vi "PH_Beamline.PC _Picture Condition Services.vi"(0 "i ref in":refnum<vi>, 2 "Instancename":string, 3 "No Link?":bool, 5 "error IO":errorcluster) -> (14 "i ref out":refnum<vi>, 19 "error out":errorcluster)   [LabVIEW 2014, in "PH_Beamline.lvlib"]
doc: "This is a Proc Case of the Beamline Class."
uses:
  PH_Beamline.lvlib
  PH_Beamline.Switch+6P Instances.ctl
  PH_Basics/PH_Common/Picture/PH_Picture.Alignment.ctl
  PH_Basics/PH_Common/Picture/PH_Picture.Size.ctl
  CS_Core/CSSystem/CSSystemLib/CSSystemLib.lvlib
  PH_Basics/PH_Beamline_Common/PH_Beamline_Common.lvlib
  PH_Basics/PH_Common/PH_Common.lvlib
  PH_BL-Master/PH_BL-Master.lvlib
panel:
  in  "Switch and 6P Instances":T1="MA01_CH1"
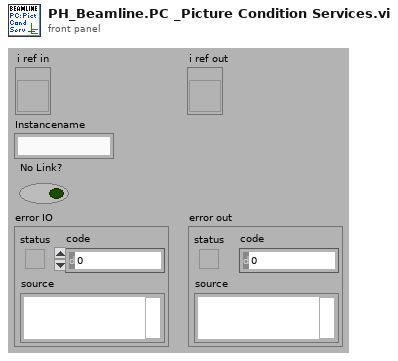
[diagram p1: front panel]
types:
  T1 = typedef "PH_Beamline.lvlib/PH_Beamline.Switch+6P Instances.ctl" = string
  T2 = typedef "PH_BL-Master.lvlib/PH_BL-Master.i attribute.ctl" = cluster{"Remote controlled":bool, "Boolean Condition Service Subscriber":refnum<vi>[], "Picture Condition Service Subscriber":refnum<vi>[], "R2S":cluster{"GUI Ref":refnum<vi>, "State":bool}, "Vacua":cluster{"GUI Ref":refnum<vi>, "Limit":dbl, "Curr Value":dbl, "in range":bool}[], "O2 Inspection":cluster{"GUI Ref":refnum<vi>, "Concentration":dbl, "State":T3}[], "Boolean Status Service Subscriber":cluster{"GUI Ref":refnum<vi>, "Status":T3, "no Link?":bool, "Status Subscriber Class":T4}[], "Picture Status Service Subscriber":cluster{"GUI Ref":refnum<vi>, "Status":T3, "no Link?":bool, "Status Subscriber Class":T4}[], "6P 4Q Service Subscriber":cluster{"GUI Ref":refnum<vi>, "Selector":T5, "no Link?":bool}[], "Index of latest 6P 4Q changing Instance":i32, "Index of latest Picture Status changing Instance":i32, "Index of latest Boolean Status changing Instance":i32, "Vision ID on same Node":string, "Start Phase over?":bool, "GUI Ref Delete":refnum<vi>}
  T3 = typedef "PH_StatusHandler.lvlib/PH_StatusHandler.Status.ctl" = i16
  T4 = typedef "PH_BL-Master.lvlib/PH_BL-Master.Status Subscriber Class.ctl" = enum16{"unknown", "Switch", "BB", "6P Switch", "Switch GUI", "Switch and 6P State", "Force Sensor"}
  T5 = typedef "PH_4_Pos_Selector.lvlib/PH_4_Pos_Selector.Position Selector.ctl" = u16
  T6 = typedef "PH_Common.lvlib/PH_Picture.Alignment.ctl" = enum16{"neutral", "left", "right", "up", "down", "vertical", "horizontal", "left down to right up", "left up to right down"}
  T7 = typedef "PH_Common.lvlib/PH_Picture.Size.ctl" = enum16{"36x36", "48x48", "24x36", "36x24", "12x60", "60x12"}
  T8 = typedef "PH_Beamline.lvlib/PH_Beamline.i attribute.ctl" = cluster{"GUI Refs":cluster{"PA ok":refnum<vi>, "MA ok":refnum<vi>, "fs FE ok":refnum<vi>, "ns FE ok":refnum<vi>, "PA ED ok":refnum<vi>, "MAS ok":refnum<vi>, "Booster ok":refnum<vi>, "Mirrortower ok":refnum<vi>, "In.-Box ok":refnum<vi>, "Compressor ok":refnum<vi>, "Experiment LB ok":refnum<vi>, "Experiment LL ok":refnum<vi>, "PHELIX_Beckhoff_Watchdog":refnum<vi>, "Shutters closed":refnum<vi>, "uOPA ok":refnum<vi>, "Vacuum no shotcond Comp LB":refnum<vi>}, "Refs BL MA":refnum<vi>[], "Refs BL MA-IB":refnum<vi>[], "Refs BL fs":refnum<vi>[], "Refs BL PA ED":refnum<vi>[], "Refs BL MAS":refnum<vi>[], "Refs BL Boo":refnum<vi>[], "Refs BL ns":refnum<vi>[], "Refs BL Mirrortower":refnum<vi>[], "Refs BL Compressor":refnum<vi>[], "Refs BL Exp LB":refnum<vi>[], "Radiation Safety":cluster{"Exp Laserbay":cluster{"Ref Op Mode":refnum<vi>, "Ref Laserbay evacuated":refnum<vi>, "Tagname LB evacuated":string, "Shot Mode":T9, "Laserbay evacuated?":i32, "Tagname HV room locked":string, "HV room locked?":i32, "Ref HV room locked":refnum<vi>, "Tagname bridged?":string, "Ref Bridge":refnum<vi>, "I<1E18W/cm²":bool}, "Exp Laserlab":cluster{"Ref Op Mode":refnum<vi>, "Ref Laserlab evacuated":refnum<vi>, "Tagname LL evacuated":string, "Shot Mode":T9, "Laserlab evacuated?":i32, "Tagname bridged?":string, "Ref Bridge":refnum<vi>, "I<1E18W/cm²":bool}}, "Refs BL LL":refnum<vi>[], "PP Igni Heating GUI Refs":refnum<vi>[], "PP Igni Heating Tagnames ":string[], "Refs BL PA":cluster{"undelayed Line before Shutter":refnum<vi>[], "undelayed Line after Shutter":refnum<vi>[], "before Bypass":refnum<vi>[], "delayed Line before Shutter":refnum<vi>[], "delayed Line after Shutter":refnum<vi>[], "before Shutter Input":refnum<vi>[], "after Shutter Input":refnum<vi>[], "Bypass":refnum<vi>[], "before Shutter Exit":refnum<vi>[], "after Shutter Exit":refnum<vi>[], "to MA":refnum<vi>[], "to Lab":refnum<vi>[]}, "BL":cluster{"YLF_BL_Status":i32, "fs_BL_Status":i32, "fs_YLF_BL_Status":i32, "ns_BL_Status":i32, "PA_Input_BL_Status":i32, "PA_UnDelay_BL_Status":i32, "PA_Delay_BL_Status":i32, "PA_BL_Status":i32, "PA_Bypass_BL_Status":i32, "PA_Exit_BL_Status":i32, "PA_LL_BL_Status":i32, "LL_BL_Status":i32, "PA_MA_BL_Status":i32, "MA_Exit_BL_Status":i32, "MA_Z6_BL_Status":i32, "Z6_BL_Status":i32, "MA_LB_BL_Status":i32, "LB_TB2_BL_Status":i32, "PA_before_Bypass_BL_Status":i32, "LB_TB3_BL_Status":i32}, "State Subsystems":cluster{"PA":bool, "MA":bool, "ns FE":bool, "fs FE":bool, "PA ED":bool, "In.-Box":bool, "MAS":bool, "Booster":bool, "Mirrortower":bool, "Compressor":bool, "Experiment LB":bool, "Experiment LL":bool, "uOPA":bool}, "Status Subscriber Information":T10, "Refs BL uOPA":refnum<vi>[], "PA_Input_2_Beam_6PWpGUI not linked?":bool, "PA_Input_Delay_6PGUI not linked?":bool, "Settings":T13}
  T9 = typedef "PH_Beamline.lvlib/PH_Beamline.Operation Mode.ctl" = i32
  T10 = typedef "PH_Beamline.lvlib/PH_Beamline.Status Subscriber Information.ctl" = cluster{"fs Swich YLF":T11, "fs Exit Shutter":T11, "ns Exit Shutter":T11, "PA Input Shutter":T11, "PA PC WP":T11, "PA PC WP 2":T11, "PA Bypass In":T11, "PA Bypass Out":T11, "PA CH 1":T11, "PA delayed":T11, "PA non delayed":T11, "PA Exit Shutter":T11, "PA Switch Lab":T11, "PA Bridge CH Input MA":T11, "MA Diffusor IB":T11, "MA IB Ready":T11, "MA CH 1":T11, "MA CH 2":T11, "MA CH 3":T11, "MA CH 4":T11, "MA Shutter Align Cam":T11, "MA Position MM5":T11, "Calorimeter Switch":T11, "BL Z6 CH 9":T11, "BL Z6 Beamdump":T11, "BL Z6 Shutter":T11, "COS Sensitivity Switch":T11, "Exp LB Shutter":T11, "Exp LB TB 2":T11, "Exp LB TB 3":T11, "PA LL Input CH":T11, "PA LL Output CH":T11, "LL Comp Input Shutter":T11, "LL Comp Output Shutter":T11, "LL Comp FF Shutter":T11, "Exp LL Shutter":T11, "MA IM In IB":T11, "MA IM Out IB":T11, "MA DB In IB":T11, "MA DB Out IB":T11, "Exp LB Shutter Interlock":T11, "Exp LL Shutter Interlock":T11, "MM1 Force Sensor":T11}
  T11 = typedef "PH_BL-Master.lvlib/PH_BL-Master.Status Subscriber Information.ctl" = cluster{"Index of element":i32, "Attributeset":T12}
  T12 = typedef "PH_BL-Master.lvlib/PH_BL-Master.Attribute Set.ctl" = enum16{"Boolean Status Service Subscriber", "Picture Status Service Subscriber"}
  T13 = typedef "PH_Beamline_Chief.lvlib/PH_Beamline_Chief.Settings.ctl" = cluster{"PA Doublepass Mode":bool, "Compressor Vaccuum LB not relevant":bool, "Windowshutter TB2 not relevant":bool, "Windowshutter TB3 not relevant":bool}
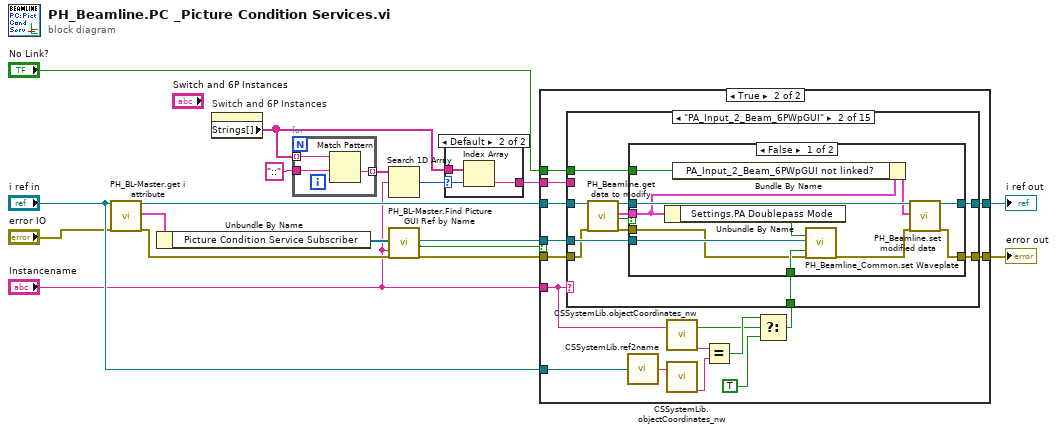
[diagram p0: block diagram]
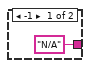
[diagram p2: hidden frame]
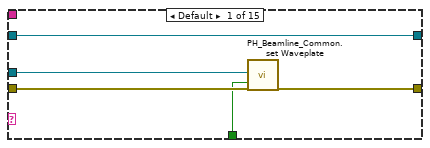
[diagram p4: hidden frame]
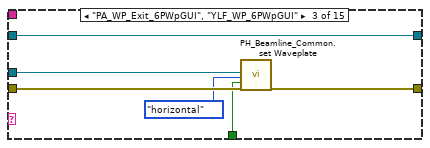
[diagram p6: hidden frame]
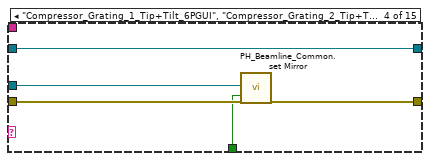
[diagram p7: hidden frame]
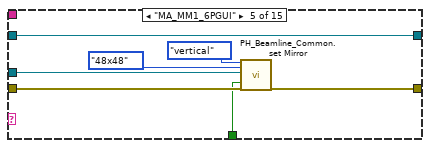
[diagram p8: hidden frame]
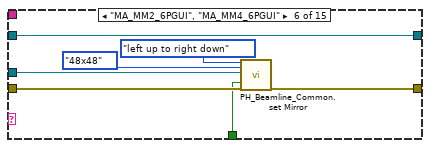
[diagram p9: hidden frame]
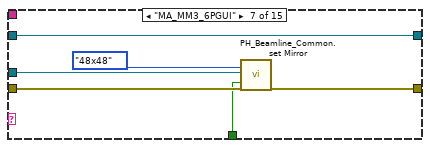
[diagram p10: hidden frame]
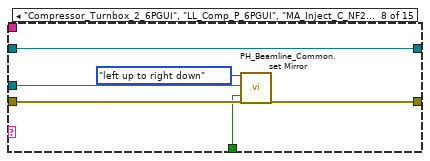
[diagram p11: hidden frame]
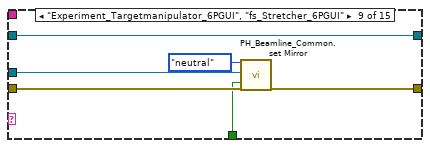
[diagram p12: hidden frame]
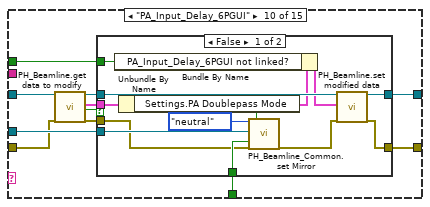
[diagram p13: hidden frame]
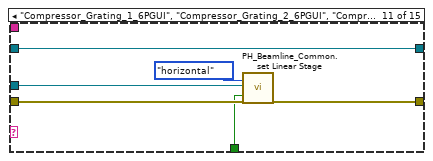
[diagram p15: hidden frame]
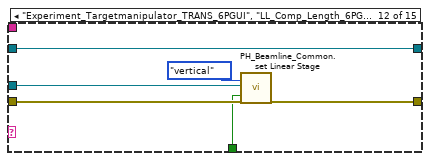
[diagram p16: hidden frame]
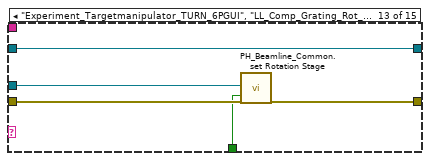
[diagram p17: hidden frame]
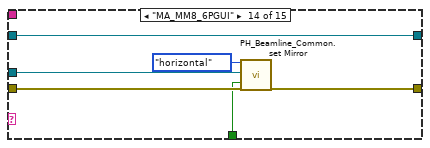
[diagram p18: hidden frame]
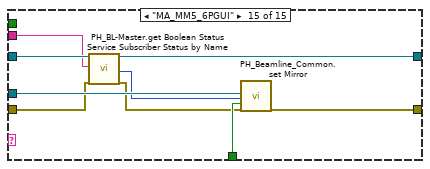
[diagram p19: hidden frame]
diagram:
  n1 = call "PH_BL-Master.get i attribute.vi"("i ref in"="i ref in", "error in (no error)"="error IO") -> ("i ref out"=w9:refnum<vi>, "i attribute"=w15:T2, "error out"=w13:errorcluster)  [unwired: 15 in]
  n2 = Unbundle By Name(w15) -> ("Picture Condition Service Subscriber"=w14:refnum<vi>[])
  n3 = property on="Switch and 6P Instances" class="CmbBox (strict)"() -> ("Strings[]"=w2:string[])  [unwired: 2 in, 2 out]
  n4 = for {
    tunnel: w2 -> [w21] mode=indexing
    tunnel: "::" ("regular expression") -> [w20]
    tunnel: [w19] -> w6 mode=indexing
    n5 = Match Pattern(string=w21, regular expression=w20) -> (after substring=w19:string)  [unwired: 1 in, 3 out]
  }
  n6 = Search 1D Array(1D array=w6, element="Instancename") -> (index of element=w4:i32)  [unwired: 1 in]
  n7 = call "PH_BL-Master.Find Picture GUI Ref by Name.vi"("Pic Ref Array"=w14, "Label"="Instancename", "error in"=w13) -> ("Wanted Pic GUI Ref"=w10:refnum<vi>, "Ref found?"=w11:bool, "error out"=w12:errorcluster)  [unwired: 13 in, 1 out]
  n8 = case shown="Default" w4 {
    selector: w4 -> [_ w24]
    tunnel: w2 -> [_ w25]
    tunnel: ["N/A" w23] -> w3
    frame -1 {
    }
    frame Default {
      n9 = Index Array(array=w25, index=w24) -> (element=w23:string)
    }
  }
  n10 = case shown="True" w11 {
    tunnel: w12 -> [w27 w35]
    tunnel: [w27 w34] -> w17
    tunnel: "Instancename" -> [_ w36]
    tunnel: "i ref in" -> [_ w43]
    tunnel: w10 -> [_ w33]
    tunnel: w9 -> [w26 w31]
    tunnel: [w26 w30] -> w8
    tunnel: w3 -> [_ w29]
    tunnel: "No Link?" -> [_ w28]
    frame False {
    }
    frame True {
      n11 = call "CSSystemLib.ref2name.vi"("obj refnum"=w43) -> ("name"=w42:string)
      n12 = call "CSSystemLib.objectCoordinates_nw.vi"("name"=w36) -> ("obj exists"=w37:bool, "node"=w38:string)  [unwired: 15 in, 2 out]
      n13 = call "CSSystemLib.objectCoordinates_nw.vi"("name"=w42) -> ("node"=w39:string)  [unwired: 15 in, 3 out]
      n14 = Equal?(x=w38, y=w39) -> (x = y?=w40:bool)
      n15 = Select(t=w40, s=w37, f=TRUE) -> (s? t:f=w32:bool)
      n16 = case shown="\"PA_Input_2_Beam_6PWpGUI\"" w36 {
        tunnel: w35 -> [w47 w55 w78 w83 w90 w97 w103 w109 w115 w122 w146 w152 w157 w163 w168]
        tunnel: [w46 w52 w77 w82 w89 w96 w102 w108 w114 w119 w145 w151 w156 w162 w172] -> w34
        tunnel: w33 -> [w48 w59 w76 w81 w88 w95 w101 w107 w113 w126 w144 w150 w155 w161 w171]
        tunnel: w32 -> [w45 w58 w75 w80 w87 w94 w100 w106 w112 w125 w143 w149 w154 w160 w170]
        tunnel: w31 -> [w44 w57 w73 w79 w84 w91 w98 w104 w110 w124 w141 w147 w153 w158 w169]
        tunnel: [w44 w53 w73 w79 w84 w91 w98 w104 w110 w120 w141 w147 w153 w158 w166] -> w30
        tunnel: w29 -> [_ _ _ _ _ _ _ _ _ _ _ _ _ _ w164]
        tunnel: w28 -> [_ w50 _ _ _ _ _ _ _ w116 _ _ _ _ _]
        frame Default {
          n17 = call "PH_Beamline_Common.set Waveplate.vi"("CtlRef"=w48, "GUI Instance does not exist or here?"=w45, "error in (no error)"=w47) -> ("error out"=w46:errorcluster)  [unwired: 16 in]
        }
        frame "PA_Input_2_Beam_6PWpGUI" {
          n18 = call "PH_Beamline.get data to modify.vi"("i ref in"=w57, "error in (no error)"=w55) -> ("i ref out"=w56:refnum<vi>, "i attribute"=w51:T8, "timed out"=w49:bool, "error out"=w54:errorcluster)  [unwired: 14 in]
          n19 = case shown="False" w49 {
            tunnel: w59 -> [w70 _]
            tunnel: w58 -> [w69 _]
            tunnel: w56 -> [w68 w72]
            tunnel: w54 -> [w67 w71]
            tunnel: [w65 w72] -> w53
            tunnel: [w63 w71] -> w52
            tunnel: w51 -> [w62 _]
            tunnel: w50 -> [w60 _]
            frame False {
              n20 = Unbundle By Name(w62) -> ("Settings.PA Doublepass Mode"=w66:bool)
              n21 = Bundle By Name(cluster=w62, "PA_Input_2_Beam_6PWpGUI not linked?"=w60) -> (w61:T8)
              n22 = call "PH_Beamline_Common.set Waveplate.vi"("Visible (true)"=w66, "CtlRef"=w70, "GUI Instance does not exist or here?"=w69, "error in (no error)"=w67) -> ("error out"=w64:errorcluster)  [unwired: 15 in]
              n23 = call "PH_Beamline.set modified data.vi"("i ref in"=w68, "i attribute"=w61, "error in (no error)"=w64) -> ("i ref out"=w65:refnum<vi>, "error out"=w63:errorcluster)  [unwired: 15 in]
            }
            frame True {
            }
          }
        }
        frame "PA_WP_Exit_6PWpGUI", "YLF_WP_6PWpGUI" {
          n24 = call "PH_Beamline_Common.set Waveplate.vi"("CtlRef"=w76, "Alignment (vertical)"=PH_Picture.Alignment."horizontal", "GUI Instance does not exist or here?"=w75, "error in (no error)"=w78) -> ("error out"=w77:errorcluster)  [unwired: 15 in]
        }
        frame "Compressor_Grating_1_Tip+Tilt_6PGUI", "Compressor_Grating_2_Tip+Tilt_6PGUI", "Compressor_LM_6PGUI", "Compressor_Turnbox_1_6PGUI", "LL_Comp_C_6PGUI", "MA_Inject_P_6PGUI", "MA_MM9_6PGUI", "PA_MM_P_Input_NF2GUI", "fs_RR_Cavity_NF2GUI" {
          n25 = call "PH_Beamline_Common.set Mirror.vi"("CtlRef"=w81, "GUI Instance does not exist or here?"=w80, "error in (no error)"=w83) -> ("error out"=w82:errorcluster)  [unwired: 16 in]
        }
        frame "MA_MM1_6PGUI" {
          n26 = call "PH_Beamline_Common.set Mirror.vi"("Alignment (left down to right up)"=PH_Picture.Alignment."vertical", "Size (36x36)"=PH_Picture.Size."48x48", "CtlRef"=w88, "GUI Instance does not exist or here?"=w87, "error in (no error)"=w90) -> ("error out"=w89:errorcluster)  [unwired: 14 in]
        }
        frame "MA_MM2_6PGUI", "MA_MM4_6PGUI" {
          n27 = call "PH_Beamline_Common.set Mirror.vi"("Alignment (left down to right up)"=PH_Picture.Alignment."left up to right down", "Size (36x36)"=PH_Picture.Size."48x48", "CtlRef"=w95, "GUI Instance does not exist or here?"=w94, "error in (no error)"=w97) -> ("error out"=w96:errorcluster)  [unwired: 14 in]
        }
        frame "MA_MM3_6PGUI" {
          n28 = call "PH_Beamline_Common.set Mirror.vi"("Size (36x36)"=PH_Picture.Size."48x48", "CtlRef"=w101, "GUI Instance does not exist or here?"=w100, "error in (no error)"=w103) -> ("error out"=w102:errorcluster)  [unwired: 15 in]
        }
        frame "Compressor_Turnbox_2_6PGUI", "LL_Comp_P_6PGUI", "MA_Inject_C_NF2GUI", "PA_C_MA_6PGUI", "PA_LL_C_6PGUI", "PA_LL_P_6PGUI", "PA_MM_C_Input_NF2GUI" {
          n29 = call "PH_Beamline_Common.set Mirror.vi"("Alignment (left down to right up)"=PH_Picture.Alignment."left up to right down", "CtlRef"=w107, "GUI Instance does not exist or here?"=w106, "error in (no error)"=w109) -> ("error out"=w108:errorcluster)  [unwired: 15 in]
        }
        frame "Experiment_Targetmanipulator_6PGUI", "fs_Stretcher_6PGUI" {
          n30 = call "PH_Beamline_Common.set Mirror.vi"("Alignment (left down to right up)"=PH_Picture.Alignment."neutral", "CtlRef"=w113, "GUI Instance does not exist or here?"=w112, "error in (no error)"=w115) -> ("error out"=w114:errorcluster)  [unwired: 15 in]
        }
        frame "PA_Input_Delay_6PGUI" {
          n31 = call "PH_Beamline.get data to modify.vi"("i ref in"=w124, "error in (no error)"=w122) -> ("i ref out"=w123:refnum<vi>, "i attribute"=w118:T8, "timed out"=w117:bool, "error out"=w121:errorcluster)  [unwired: 14 in]
          n32 = case shown="False" w117 {
            tunnel: w126 -> [w138 _]
            tunnel: w125 -> [w137 _]
            tunnel: w123 -> [w135 w140]
            tunnel: w121 -> [w134 w139]
            tunnel: [w132 w140] -> w120
            tunnel: [w130 w139] -> w119
            tunnel: w118 -> [w129 _]
            tunnel: w116 -> [w127 _]
            frame False {
              n33 = Bundle By Name(cluster=w129, "PA_Input_Delay_6PGUI not linked?"=w127) -> (w128:T8)
              n34 = Unbundle By Name(w129) -> ("Settings.PA Doublepass Mode"=w133:bool)
              n35 = call "PH_Beamline_Common.set Mirror.vi"("Alignment (left down to right up)"=PH_Picture.Alignment."neutral", "CtlRef"=w138, "GUI Instance does not exist or here?"=w137, "error in (no error)"=w134, "Visible (true)"=w133) -> ("error out"=w131:errorcluster)  [unwired: 14 in]
              n36 = call "PH_Beamline.set modified data.vi"("i ref in"=w135, "i attribute"=w128, "error in (no error)"=w131) -> ("i ref out"=w132:refnum<vi>, "error out"=w130:errorcluster)  [unwired: 15 in]
            }
            frame True {
            }
          }
        }
        frame "Compressor_Grating_1_6PGUI", "Compressor_Grating_2_6PGUI", "Compressor_Turnbox_1_Trans_6PGUI", "Compressor_Turnbox_2_Trans_6PGUI" {
          n37 = call "PH_Beamline_Common.set Linear Stage.vi"("Alignment (vertical)"=PH_Picture.Alignment."horizontal" ("Alignment (left down to right up)"), "CtlRef"=w144, "GUI Instance does not exist or here?"=w143, "error in (no error)"=w146) -> ("error out"=w145:errorcluster)  [unwired: 15 in]
        }
        frame "Experiment_Targetmanipulator_TRANS_6PGUI", "LL_Comp_Length_6PGUI" {
          n38 = call "PH_Beamline_Common.set Linear Stage.vi"("Alignment (vertical)"=PH_Picture.Alignment."vertical" ("Alignment (left down to right up)"), "CtlRef"=w150, "GUI Instance does not exist or here?"=w149, "error in (no error)"=w152) -> ("error out"=w151:errorcluster)  [unwired: 15 in]
        }
        frame "Experiment_Targetmanipulator_TURN_6PGUI", "LL_Comp_Grating_Rot_6PGUI" {
          n39 = call "PH_Beamline_Common.set Rotation Stage.vi"("CtlRef"=w155, "GUI Instance does not exist or here?"=w154, "error in (no error)"=w157) -> ("error out"=w156:errorcluster)  [unwired: 16 in]
        }
        frame "MA_MM8_6PGUI" {
          n40 = call "PH_Beamline_Common.set Mirror.vi"("Alignment (left down to right up)"=PH_Picture.Alignment."horizontal", "CtlRef"=w161, "GUI Instance does not exist or here?"=w160, "error in (no error)"=w163) -> ("error out"=w162:errorcluster)  [unwired: 15 in]
        }
        frame "MA_MM5_6PGUI" {
          n41 = call "PH_BL-Master.get Boolean Status Service Subscriber Status by Name.vi"("i ref in"=w169, "Status Subscriber Instance"=w164, "error in (no error)"=w168) -> ("i ref out"=w166:refnum<vi>, "Subscriber State"=w165:T3, "error out"=w167:errorcluster)  [unwired: 7 in, 7 out]
          n42 = call "PH_Beamline_Common.set Mirror.vi"("CtlRef"=w171, "Status (on/true/in)"=w165, "GUI Instance does not exist or here?"=w170, "error in (no error)"=w167) -> ("error out"=w172:errorcluster)  [unwired: 15 in]
        }
      }
    }
  }
  "error out" <- w17
  "i ref out" <- w8
